vi "ToString.vi"(8 "error in (no error)":errorcluster, 11 "Fact in":refnum<class "Fact.lvclass">) -> (0 "error out":errorcluster, 2 "String":string, 3 "Fact out":refnum<class "Fact.lvclass">)   [LabVIEW 2019, in "TestCase.lvlib" / "Fact.lvclass"]
doc: "Returns the string representation for this object."
uses:
  Fact.lvclass
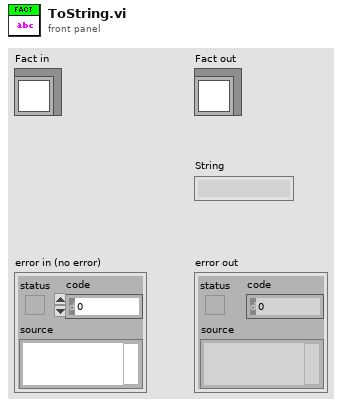
[diagram p1: front panel]
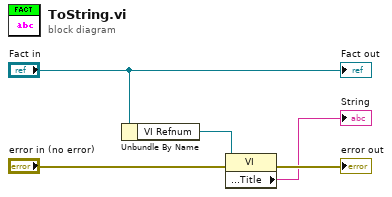
[diagram p0: block diagram]
diagram:
  n1 = Unbundle By Name("Fact in") -> ("VI Refnum"=w2:refnum<vi>)
  n2 = property class="VI"(reference=w2, error in="error in (no error)") -> (error out=→"error out":errorcluster, "Front Panel.Title"=→"String":string)  [unwired: 1 out]
  "Fact out" <- "Fact in"
